vi "FTW-Endpoint-ConnectToListener.vi"(0 "FTW-Endpoint In":refnum<class "FTW-Endpoint.lvclass">, 5 "Address":string, 9 "Timeout":i32=1000 format="%dmsec", 11 "error in":errorcluster) -> (4 "FTW-Endpoint Out":refnum<class "FTW-Endpoint.lvclass">, 6 "Actual Address":string, 15 "error out":errorcluster)   [LabVIEW 2013, in "FTW-Endpoint.lvclass"]
uses:
  FTW-Endpoint.lvclass
  FTW-Endpoint.lvclass/FTW-Endpoint.ctl
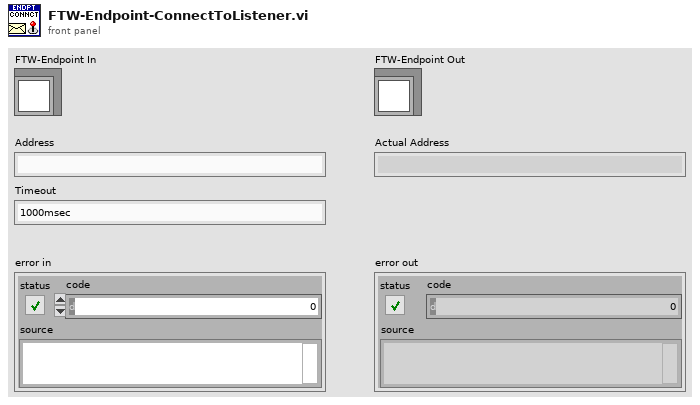
[diagram p1: front panel]
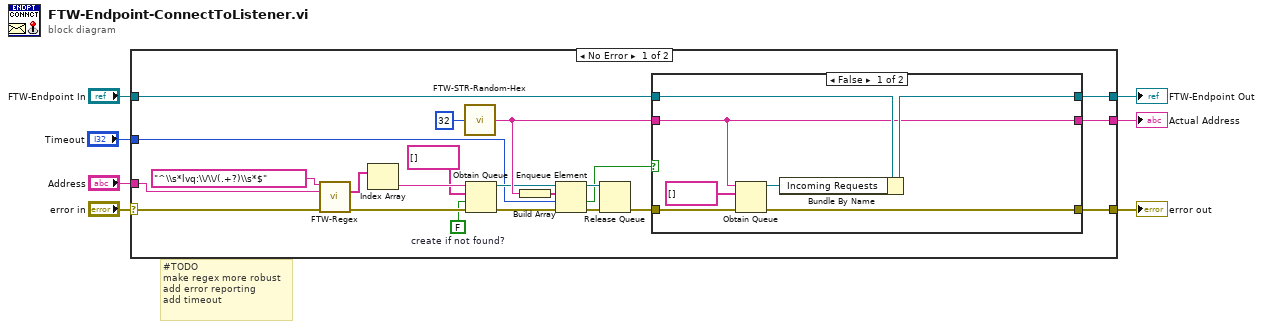
[diagram p0: block diagram]
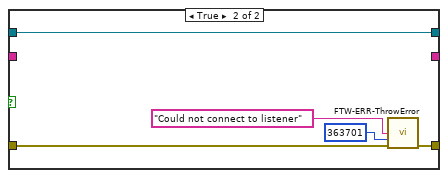
[diagram p2: hidden frame]
diagram:
  # "#TODO\nmake regex more robust\nadd error reporting\nadd timeout"
  n1 = case shown="No Error" "error in" {
    selector: "error in" -> [w27 w43]
    tunnel: [w23 w43] -> w7
    tunnel: [w22 w42] -> w6
    tunnel: "FTW-Endpoint In" -> [w28 w42]
    tunnel: "Address" -> [w19 _]
    tunnel: [w20 _] -> w2
    tunnel: "Timeout" -> [w11 _]
    frame No Error {
      w13 = FALSE  # create if not found?
      n2 = call "FTW-Regex.vi"("Regular Expression"="^\\s*lvq:\\/\\/(.+?)\\s*$" ("input string"), "Input String"=w19, "error in"=w27) -> ("Submatches"=w25:string[], "error out"=w26:errorcluster)  [unwired: 8 in, 3 out]
      n3 = Index Array(array=w25) -> (element=w24:string)  [unwired: 1 in]
      n4 = call "FTW-STR-Random-Hex.vi"("String Length"=32) -> ("Random Hex String"=w21:string)  [unwired: 3 in]
      n5 = Obtain Queue(name (unnamed)=w24, element data type=string[] [], create if not found? (T)=w13, error in (no error)=w26) -> (queue out=w15:refnum<queue>, error out=w17:errorcluster)  [unwired: 1 in, 1 out]
      n6 = Build Array(w21) -> (w9:string[])
      n7 = Enqueue Element(queue=w15, element=w9, timeout in ms (-1)=w11, error in (no error)=w17) -> (queue out=w14:refnum<queue>, timed out?=w10:bool, error out=w16:errorcluster)
      n8 = Release Queue(queue=w14, error in (no error)=w16) -> (error out=w29:errorcluster)  [unwired: 1 in, 2 out]
      n9 = case shown="False" w10 {
        tunnel: w29 -> [w36 w40]
        tunnel: w28 -> [w35 w41]
        tunnel: [w33 w39] -> w23
        tunnel: [w34 w41] -> w22
        tunnel: w21 -> [w31 _]
        tunnel: [w31 _] -> w20
        frame False {
          n10 = Obtain Queue(name (unnamed)=w31, element data type=string[] [], error in (no error)=w36) -> (queue out=w32:refnum<queue>, error out=w33:errorcluster)  [unwired: 2 in, 1 out]
          n11 = Bundle By Name(cluster=w35, "Incoming Requests"=w32) -> (w34:refnum<class "FTW-Endpoint.lvclass">)
        }
        frame True {
          n12 = call "FTW-ERR-ThrowError.vi"("Error Message"="Could not connect to listener", "Error Code"=363701, "error in"=w40) -> ("error out"=w39:errorcluster)  [unwired: 12 in]
        }
      }
    }
    frame Error {
    }
  }
  "FTW-Endpoint Out" <- w6
  "error out" <- w7
  "Actual Address" <- w2
